vi "Calcul Offset_XY.vi"(2 "Rot(rad)":dbl format="%.2f", 3 "Arcmin/pulse":dbl format="%.2f", 4 "offset DEC":dbl format="%.2f", 5 "offset RA":dbl format="%.2f") -> (0 "X":i32, 1 "Y":i32)   [LabVIEW 2011]
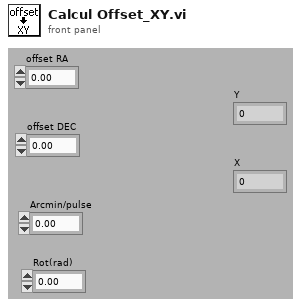
[diagram p1: front panel]
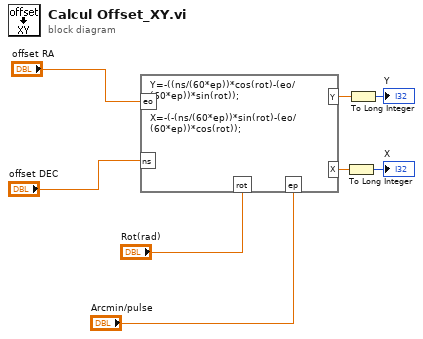
[diagram p0: block diagram]
diagram:
  n1 = formula code="Y=-((ns/(60*ep))*cos(rot)-(eo/(60*ep))*sin(rot));\n\nX=-(-(ns/(60*ep))*sin(rot)-(eo/(60*ep))*cos(rot));"("ns"="offset DEC", "eo"="offset RA", "ep"="Arcmin/pulse", "rot"="Rot(rad)") -> ("X"=w3:dbl, "Y"=w4:dbl)
  n2 = To Long Integer(number=w3) -> (32bit integer=→"X":i32)
  n3 = To Long Integer(number=w4) -> (32bit integer=→"Y":i32)
